vi "FreqEstimator.vi"() -> ()   [LabVIEW 2014]
uses:
  <vilib>/measure/NI_MABase.lvlib
panel:
  out "Waveform Graph":waveform(dbl)(graph)
  out "Freq Error":dbl
  in  "frequency":dbl=10.0 format="%#_13g"
  in  "Estimation Model":string(combo)="power"
  in  "sampling info":cluster{"Fs":dbl, "#s":dbl}={"Fs"=1000.0, "#s"=1000.0} {"Fs" format="%.2p"}
  in  "Signal type":T1(ring)
  out "Estimated frequency":dbl format="%.7g"
  out "Signal":dbl[](array[numeric])
  out "fs":dbl=5000.0
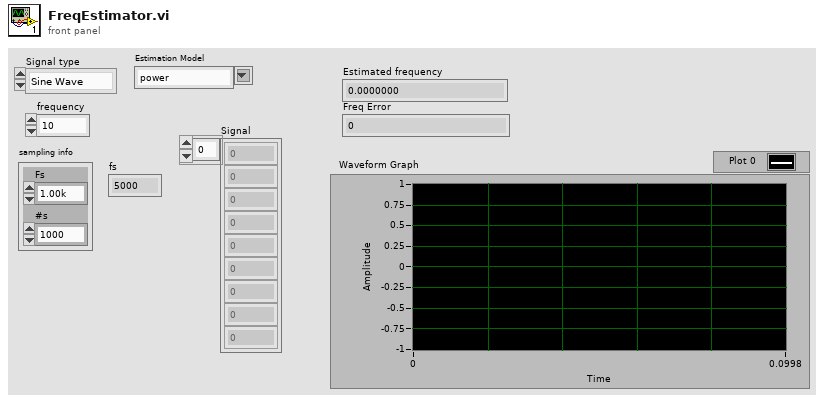
[diagram p1: front panel]
types:
  T1 = enum16{"Sine Wave", "Triangle Wave", "Square Wave", "Sawtooth Wave"}
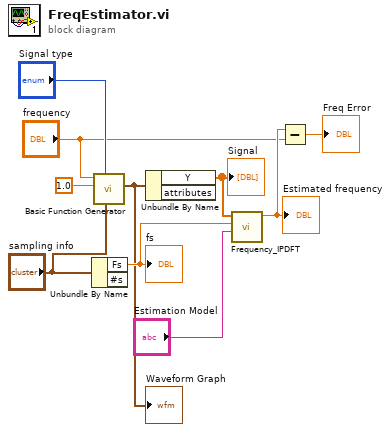
[diagram p0: block diagram]
diagram:
  n1 = Unbundle By Name("sampling info") -> ("Fs"=w5:dbl)  [unwired: 1 out]
  "fs" <- w5
  n2 = call <vilib>:"Basic Function Generator.vi"("sampling info"="sampling info", "signal type"="Signal type", "amplitude"=1.0, "frequency"="frequency") -> ("signal out"=w1:waveform(dbl))  [unwired: 5 in, 2 out]
  "Waveform Graph" <- w1
  n3 = Unbundle By Name(w1) -> ("Y"=w7:dbl[])  [unwired: 1 out]
  "Signal" <- w7
  n4 = call "Frequency_IPDFT.vi"("Estimation Model"="Estimation Model", "Fs"=w5, "Signal"=w7) -> ("f"=w4:dbl)  [unwired: 8 in]
  "Estimated frequency" <- w4
  n5 = Subtract(x=w4, y="frequency") -> (x-y=→"Freq Error":dbl)
